vi "SingleWithPayload.vi"(6 "Payload":variant, 9 "Action":string) -> (1 "ActionStack out":refnum<class "Action.lvclass">)   [LabVIEW 2024, in "ActionStack.lvlib" / "Action.lvclass"]
uses:
  Action.lvclass
  Action.lvclass/Action.ctl
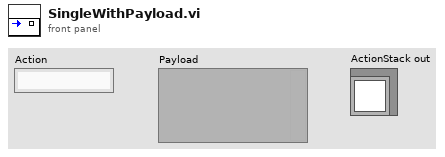
[diagram p1: front panel]
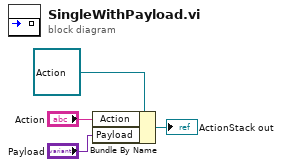
[diagram p0: block diagram]
diagram:
  n1 = Bundle By Name(cluster=refnum<class "Action.lvclass"> refnum ("ActionStack.lvclass"), "Action"="Action", "Payload"="Payload") -> (→"ActionStack out":refnum<class "Action.lvclass">)
